vi "connect.vi"(8 "error in (no error)":errorcluster, 11 "MonoClientCommunicator in":refnum<class "MonoClientCommunicator.lvclass">) -> (0 "error out":errorcluster, 3 "MonoClientCommunicator out":refnum<class "MonoClientCommunicator.lvclass">)   [LabVIEW 2016, in "MonoClientCommunicator.lvclass"]
uses:
  MonoClientCommunicator.lvclass
  MonoClientCommunicator.lvclass/MonoClientCommunicator.ctl
  ts_labview_tcp/TCPClient/TCPClient.lvclass
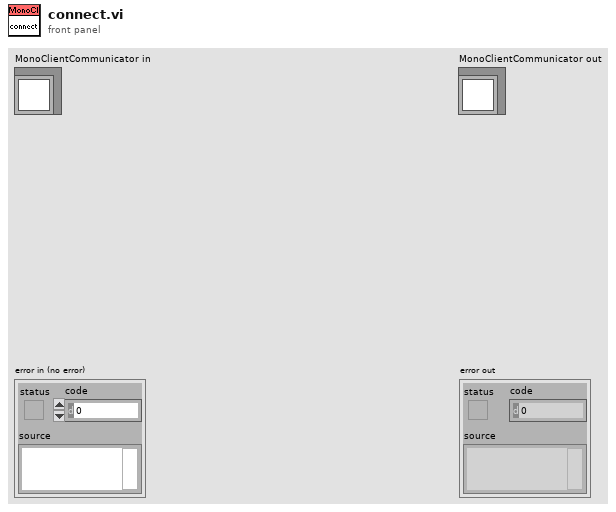
[diagram p1: front panel]
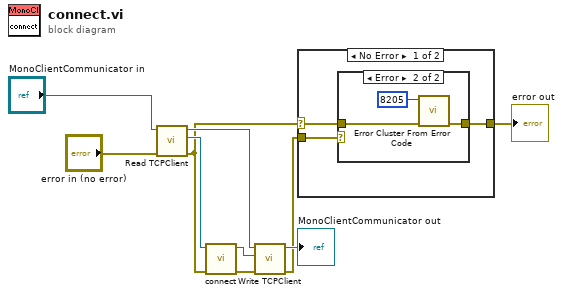
[diagram p0: block diagram]
diagram:
  n1 = call "Read TCPClient.vi"("error in (no error)"="error in (no error)", "MonoClient in"="MonoClientCommunicator in") -> ("error out"=w3:errorcluster, "TCPClient.lvclass"=w6:refnum<class "TCPClient.lvclass">, "MonoClient out"=w10:refnum<class "MonoClientCommunicator.lvclass">)  [unwired: 7 in]
  n2 = call-dynamic "connect.vi"("error in (no error)"=w3, "TCPClient in"=w6) -> ("error out"=w4:errorcluster, "TCPClient out"=w5:refnum<class "TCPClient.lvclass">)  [unwired: 8 in]
  n3 = call "Write TCPClient.vi"("error in (no error)"=w4, "TCPClient.lvclass"=w5, "MonoClient in"=w10) -> ("error out"=w1:errorcluster, "MonoClient out"=→"MonoClientCommunicator out":refnum<class "MonoClientCommunicator.lvclass">)  [unwired: 7 in]
  n4 = case shown="No Error" w3 {
    selector: w3 -> [w11 w18]
    tunnel: [w12 w18] -> w2
    tunnel: w1 -> [w13 _]
    frame No Error {
      n5 = case shown="Error" w13 {
        selector: w13 -> [w14 _]
        tunnel: [w14 w16] -> w12
        tunnel: w11 -> [_ w17]
        frame No Error {
        }
        frame Error {
          n6 = call <vilib>:"Error Cluster From Error Code.vi"("error in (no error)"=w17, "error code (0)"=8205) -> ("error out"=w16:errorcluster)  [unwired: 7 in]
        }
      }
    }
    frame Error {
    }
  }
  "error out" <- w2
